vi "Get Start Point.vi"(8 "Altitude (m)":dbl, 9 "Camera Settings":T2, 10 "Lon":dbl, 11 "Lat":dbl) -> (0 "Frame Height (m)":dbl, 1 "Frame Width (m)":dbl, 2 "Point Offset":T1 {"Latitude" format="%#_10g"; "Longitude" format="%#_10g"})   [LabVIEW 2014]
uses:
  Settings File/Controls/Camera Settings.ctl
  Lat Long Conversion/Controls/PointLatLon.ctl
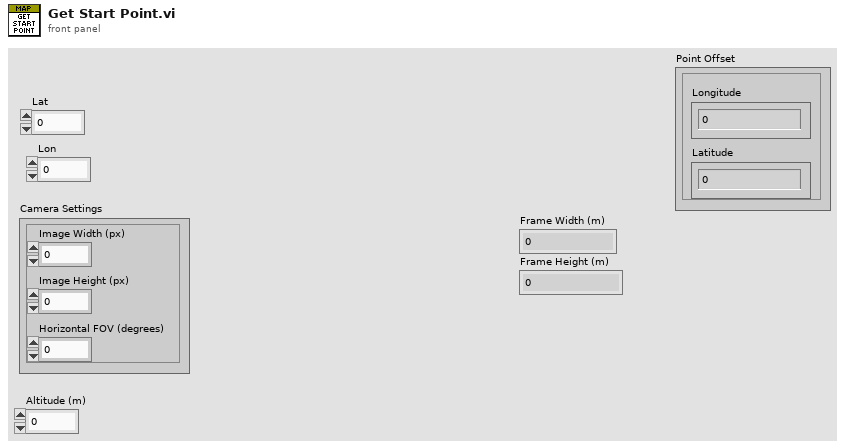
[diagram p1: front panel]
types:
  T1 = typedef "PointLatLon.ctl" = cluster{"Longitude":dbl, "Latitude":dbl}
  T2 = typedef "Camera Settings.ctl" = cluster{"Image Width (px)":dbl, "Image Height (px)":dbl, "Horizontal FOV (degrees)":dbl}
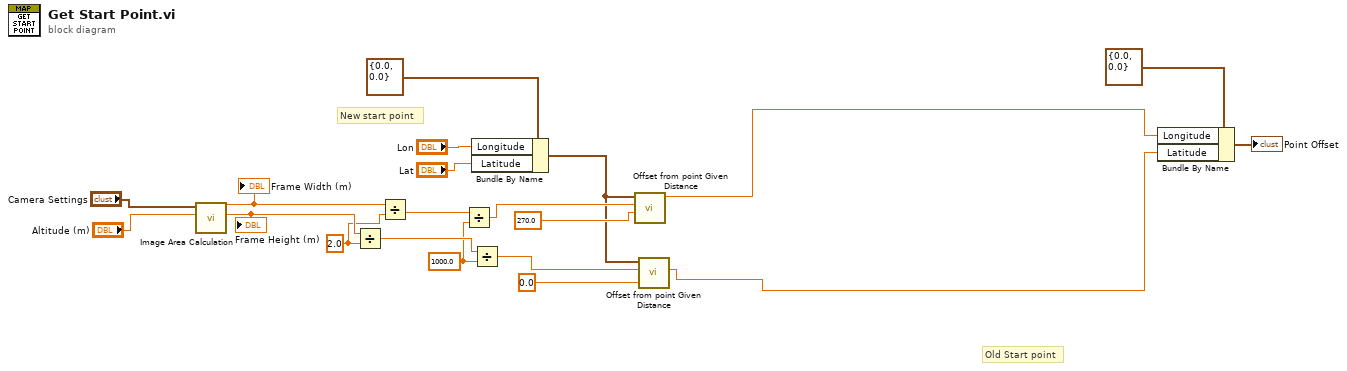
[diagram p0: block diagram]
diagram:
  w5 = 1000.0 ("y")
  w12 = 2.0 ("y")
  # "New start point"
  # "Old Start point"
  n1 = call "Image Area Calculation.vi"("Altitude (m)"="Altitude (m)", "Camera Settings"="Camera Settings") -> ("Height (m)"=w14:dbl, "Width (m)"=w13:dbl)  [unwired: 6 in, 2 out]
  "Frame Width (m)" <- w13
  "Frame Height (m)" <- w14
  n2 = Divide(x=w14, y=w12) -> (x/y=w6:dbl)
  n3 = Divide(x=w13, y=w12) -> (x/y=w7:dbl)
  n4 = Divide(x=w7, y=w5) -> (x/y=w4:dbl)
  n5 = Bundle By Name(cluster=T1 {"Longitude"=0.0, "Latitude"=0.0} ("Origin Point"), "Longitude"="Lon", "Latitude"="Lat") -> (w1:T1)
  n6 = Divide(x=w6, y=w5) -> (x/y=w3:dbl)
  n7 = call "Offset from point Given Distance.vi"("Bearing (clockwise from North)"=270.0, "Distance (km)"=w4, "Origin Point"=w1) -> ("Lon Offset"=w10:dbl)  [unwired: 5 in, 3 out]
  n8 = call "Offset from point Given Distance.vi"("Bearing (clockwise from North)"=0.0, "Distance (km)"=w3, "Origin Point"=w1) -> ("Lat Offset"=w9:dbl)  [unwired: 5 in, 3 out]
  n9 = Bundle By Name(cluster=T1 {"Longitude"=0.0, "Latitude"=0.0} ("Origin Point"), "Longitude"=w10, "Latitude"=w9) -> (→"Point Offset":T1)
